vi "Message_Splitter.vi"(10 "W2":u8[](array[numeric]), 11 "W1":u8[](array[numeric])) -> (1 "Wp2":u8[](array[numeric]), 2 "Wp1":u8[](array[numeric]), 3 "Wc":u8[](array[numeric]))   [LabVIEW 2022 SP3]
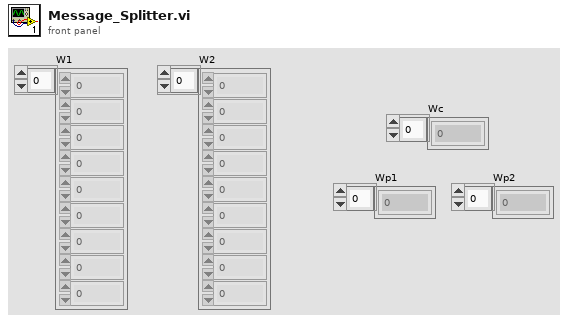
[diagram p1: front panel]
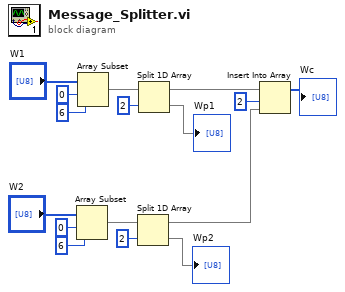
[diagram p0: block diagram]
diagram:
  n1 = Array Subset(array="W2", index=0, length=6) -> (w7:u8[])
  n2 = Array Subset(array="W1", index=0, length=6) -> (w13:u8[])
  n3 = Split 1D Array(array=w7, index=2) -> (first subarray=w3:u8[], second subarray=→"Wp2":u8[])
  n4 = Split 1D Array(array=w13, index=2) -> (first subarray=w4:u8[], second subarray=→"Wp1":u8[])
  n5 = Insert Into Array(array=w4, index=2, new element=w3) -> (→"Wc":u8[])
